vi "data_input.vi"() -> ()   [LabVIEW 2026]
uses:
  <vilib>/DAQmx/read.llb/DAQmx Read.vi
  <vilib>/DAQmx/read.llb/DAQmx Read (Analog 1D Wfm NChan NSamp).vi
  <vilib>/DAQmx/miscellaneous.llb/DAQmx Fill In Error Info.vi
  <vilib>/ptbypt/NI_PtbyPt.lvlib
panel:
  out "Numeric":dbl
  in  "stop":bool
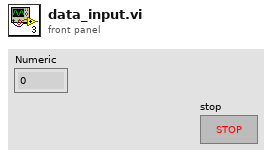
[diagram p1: front panel]
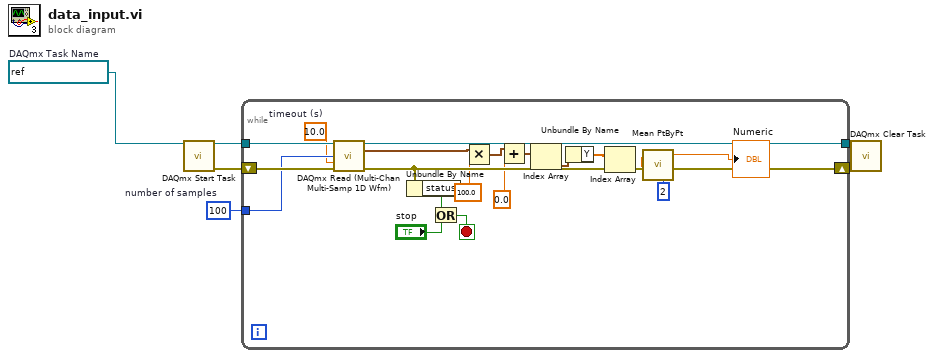
[diagram p0: block diagram]
diagram:
  w4 = 100  # number of samples
  w1 = refnum<k21> "MyVoltageTask"  # DAQmx Task Name
  n1 = call <vilib>:"DAQmx Start Task.vi"("task/channels in"=w1) -> ("task out"=w6:refnum<k21>, "error out"=w5:errorcluster)  [unwired: 13 in]
  n2 = while {
    tunnel: w6 -> [w25]
    tunnel: w4 -> [w22]
    tunnel: [w23] -> w2
    shift-right: [w20] -> w3
    shift-left: w5 -> [w24]
    stop <- w19 stop-if-true
    w17 = 10.0  # timeout (s)
    n3 = call-poly "DAQmx Read (Multi-Chan Multi-Samp 1D Wfm).vi"("task/channels in"=w25, "number of samples per channel"=w22, "timeout"=w17, "error in"=w24) -> ("task out"=w23:refnum<k21>, "data"=w14:waveform(dbl)[], "error out"=w20:errorcluster)  [unwired: 9 in]
    n4 = Unbundle By Name(w20) -> ("status"=w21:bool)
    n5 = Or(x=w21, y="stop") -> (x .or. y?=w19:bool)
    n6 = Multiply(x=w14, y=100.0) -> (x*y=w13:waveform(dbl)[])
    n7 = Add(x=w13, y=0.0) -> (x+y=w12:waveform(dbl)[])
    n8 = Index Array(array=w12) -> (element=w11:waveform(dbl))  [unwired: 1 in]
    n9 = Unbundle By Name(w11) -> ("Y"=w9:dbl[])
    n10 = Index Array(array=w9) -> (element=w8:dbl)  [unwired: 1 in]
    n11 = call <vilib>:"Mean PtByPt.vi"("x"=w8, "sample length"=2) -> ("mean"=→"Numeric":dbl)  [unwired: 2 in, 1 out]
  }
  n12 = call <vilib>:"DAQmx Clear Task.vi"("task in"=w2, "error in"=w3) -> ()  [unwired: 13 in, 1 out]
